vi "CharToAscii（U8 Array to String）.vi"(1 "Char":string) -> (0 "ASCII":u8 format="DEC:%2d\nHEX:%2x")   [LabVIEW 2012]
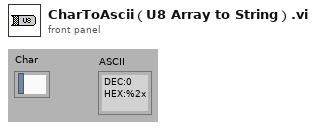
[diagram p1: front panel]
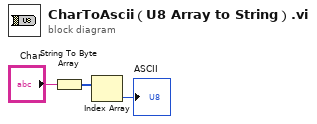
[diagram p0: block diagram]
diagram:
  n1 = String To Byte Array(string="Char") -> (unsigned byte array=w2:u8[])
  n2 = Index Array(array=w2) -> (element=→"ASCII":u8)  [unwired: 1 in]
